vi "g_Excuse_Column_Titles.vi"() -> ()   [LabVIEW 2015, in "Member_Actor.lvlib" / "ExcuseNote.lvclass"]
uses:
  ExcuseNote.lvclass
panel:
  in  "ExcuseNote_Column_Titles":string[](array[string])=["姓名", "学号", "当前周次", "请假日期", "请假开始节次", "请假结束节次", "请假理由"]
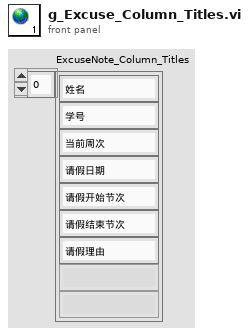
[diagram p1: front panel]
diagram:
